vi "Paint.lv.vi"() -> ()   [LabVIEW 2015]
uses:
  Buttons/Line.ctl
  Buttons/Rectangle.ctl
  Buttons/Triangle.ctl
  Buttons/Undo.ctl
  Buttons/Redo.ctl
  Buttons/Clear.ctl
  Graphic Objects/Graphic/Ctls/Style.ctl
  <vilib>/event_ctls.llb/eventvkey.ctl
  Graphic Objects/Canvas/Type Definitions/Status.ctl
  Graphic Objects/Graphic/Graphic.lvclass/Graphic.ctl
  Graphic Objects/Canvas/Canvas.lvclass/Canvas.ctl
  Graphic Objects/Canvas/Canvas.lvclass
  <vilib>/Utility/miscctls.llb/LVPoint32TypeDef.ctl
  Graphic Objects/Graphic/Graphic.lvclass
  Graphic Objects/Line/Line.lvclass
  Graphic Objects/Line Border/Line Border.lvclass
  Graphic Objects/Rectangle/Rectangle.lvclass
  Graphic Objects/Rectangle Border/Rectangle Border.lvclass
  Graphic Objects/Triangle/Triangle.lvclass
panel:
  in  "Listbox":i32(listbox)
  in  "Tool Box":enum32{"Line", "Rectangle", "Triangle"}(radio)
  in  "Clear":T1
  in  "Redo":T2
  in  "Undo":T3
  out "Border":picture
  out "Picture":picture
  in  "Line Type":T4(ring) caption="Line Type:"
  in  "Line Width":u8=2 caption="Line Width:" min=1 max=10 step=1
  in  "Line Color":u32(colorbox) caption="Line Color:"
  # "Paint.lv"
  # "V1.0.1"
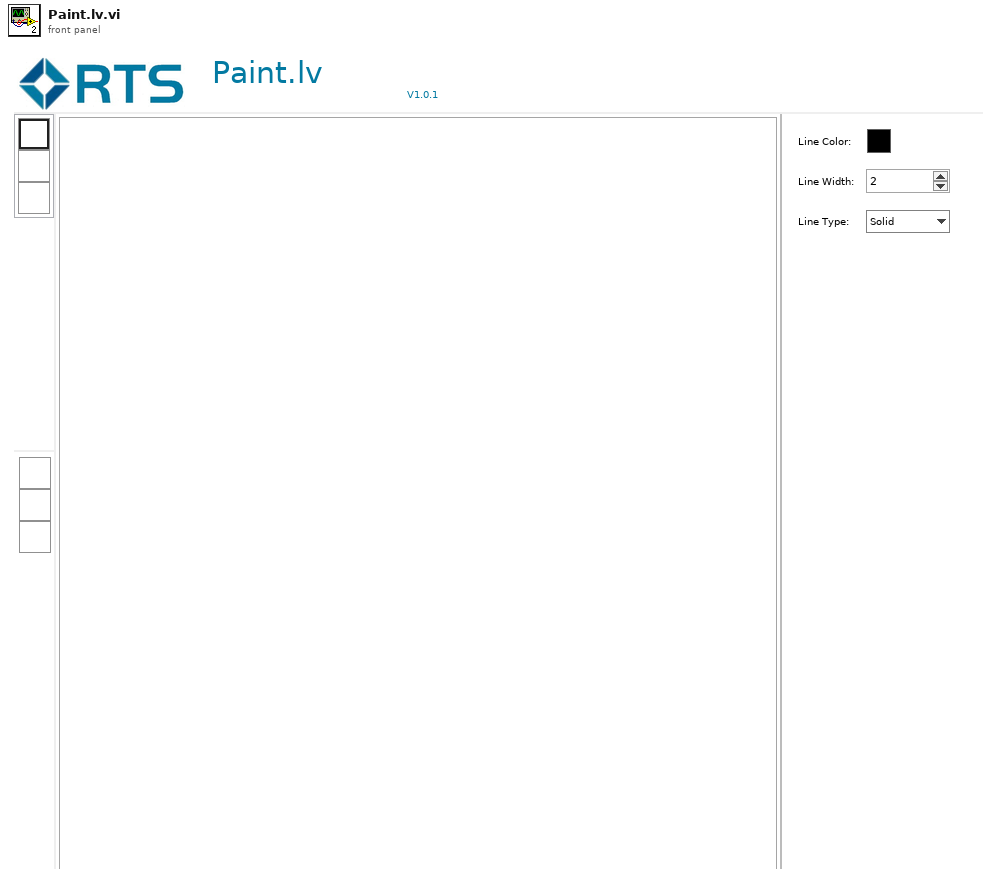
[diagram p1: front panel]
types:
  T1 = typedef "Clear.ctl" = bool
  T2 = typedef "Redo.ctl" = bool
  T3 = typedef "Undo.ctl" = bool
  T4 = enum32{"Solid", "Dash", "Dot", "DashDot", "DashDotDot"}
  T5 = typedef "Graphic.lvclass/Style.ctl" = cluster{"Color":u32, "Pen":cluster{"Width":u16, "Style":enum32{"Solid", "Dash", "Dot", "DashDot", "DashDotDot"}}}
  T6 = typedef "eventvkey.ctl" = enum16{"ASCII", "Enter", "Return", "Shift", "Ctrl", "Alt", "Cmd", "Opt", "Caps", "NumLock", "Clear", "Break", "Up", "Down", "Left", "Right", "Insert", "Delete", "Home", "End", "PageUp", "PageDown", "Escape", "Help", "Pause", "ScrollLock", "F1", "F2", "F3", "F4", "F5", "F6", "F7", "F8", "F9", "F10", "F11", "F12", "F13", "F14", "F15", "F16", "F17", "F18", "F19", "F20", "F21", "F22", "F23", "F24", "Play", "VolumeUp", "VolumeDown", "Mute", "Two Byte Char"}
  T7 = typedef "Canvas.lvclass/Status.ctl" = enum16{"Idle", "Drawing", "Modify"}
  T8 = enum32{"Invalid", "Standard", "Closed", "Hidden", "Minimized", "Maximized"}
  T9 = enum32{"invalid app kind", "Development System", "Run Time System", "Student Edition", "Embedded LabVIEW", "Evaluation", "Custom"}
  T10 = typedef "LVPoint32TypeDef.ctl" = cluster{"Horizontal":i32, "Vertical":i32}
  T11 = cluster{"Core":cluster{"Current VI Reference":refnum<vi>, "Close Panel on Exit?":bool}, "Canvas":refnum<class "Canvas.lvclass">, "MouseDown Coords":T10, "MouseUp Coords":T10, "Current Coords":T10, "Status":T7, "Drawing Graphic":refnum<class "Graphic.lvclass">, "ValidOperating":bool, "MouseDown":bool}
  T12 = cluster{"Width":u16, "Style":enum32{"Solid", "Dash", "Dot", "DashDot", "DashDotDot"}}
  T13 = cluster{"Current VI Reference":refnum<vi>, "Close Panel on Exit?":bool}
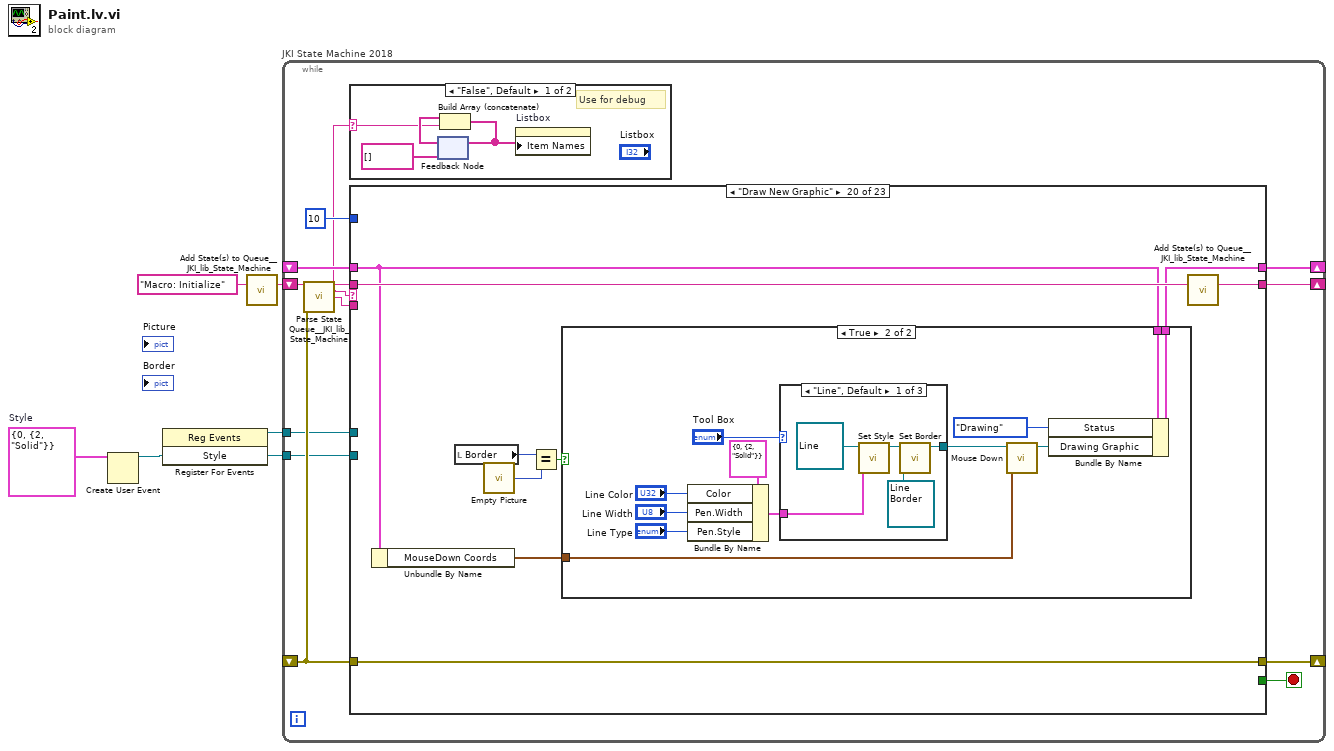
[diagram p0: block diagram]
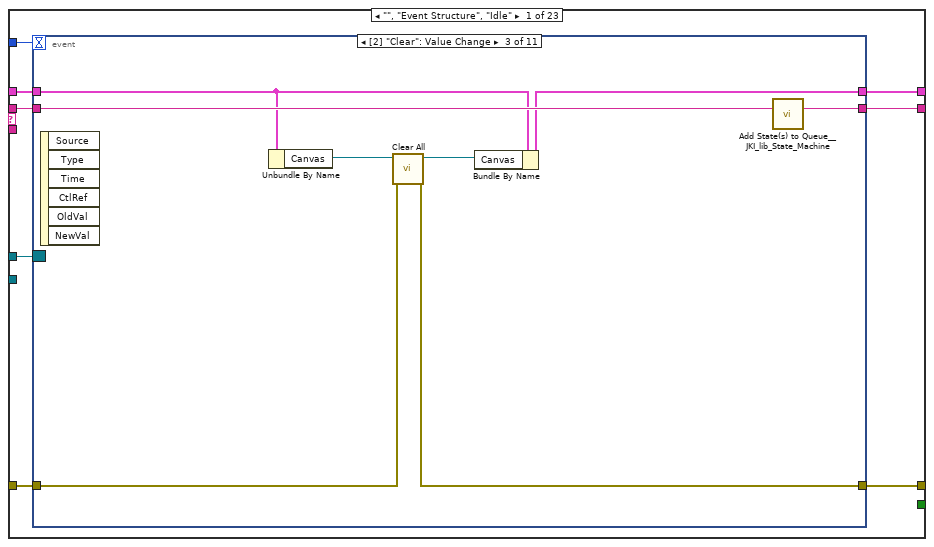
[diagram p3: hidden frame]
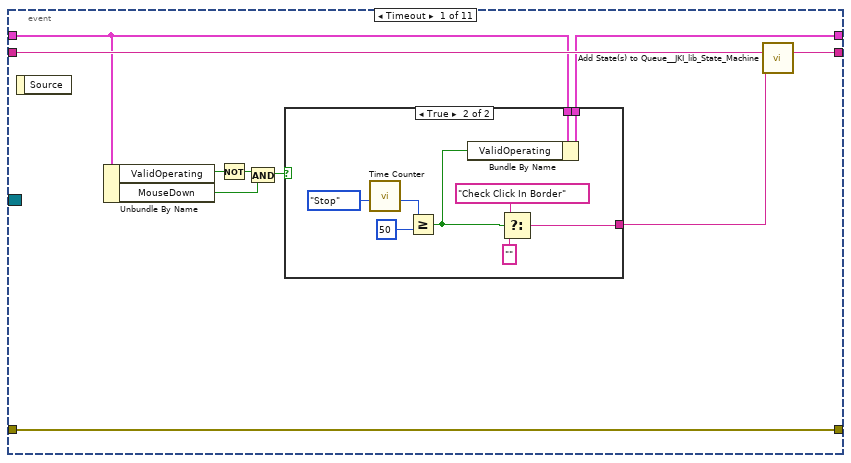
[diagram p4: hidden frame]
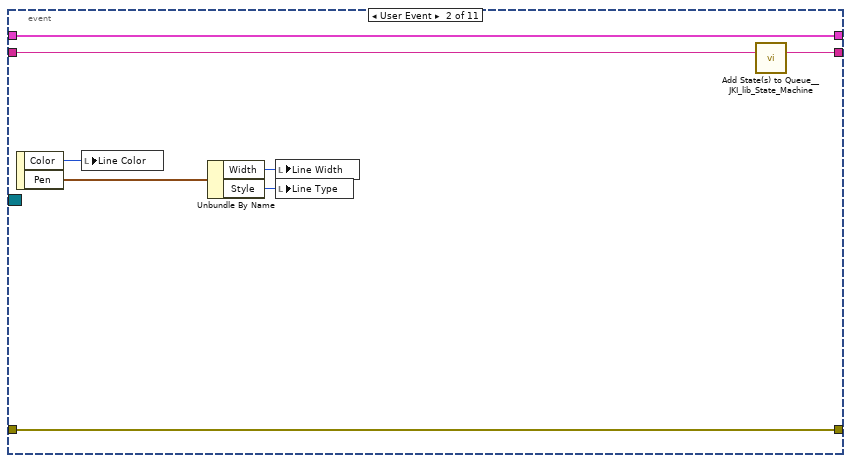
[diagram p6: hidden frame]
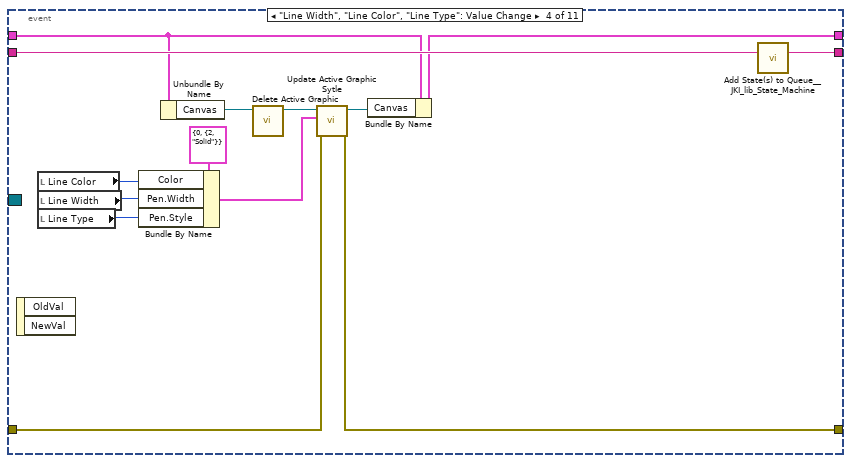
[diagram p7: hidden frame]
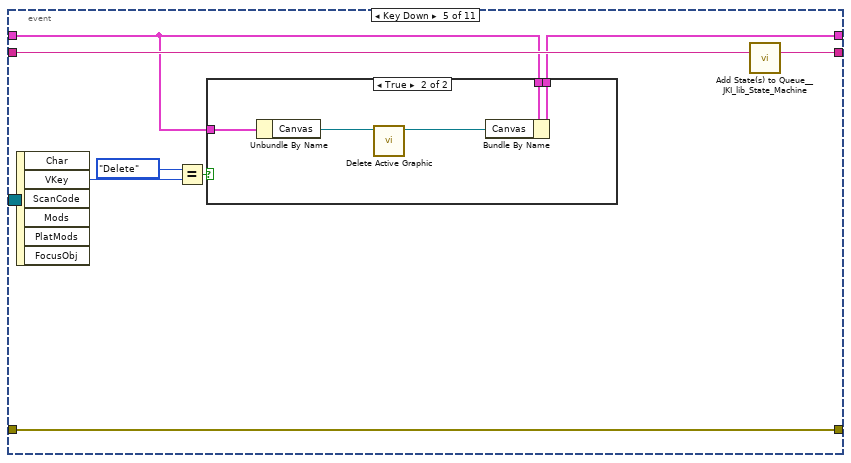
[diagram p8: hidden frame]
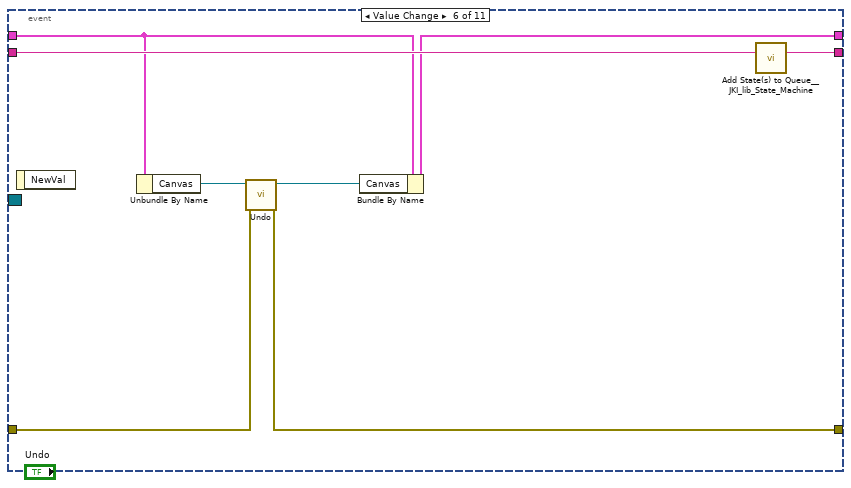
[diagram p10: hidden frame]
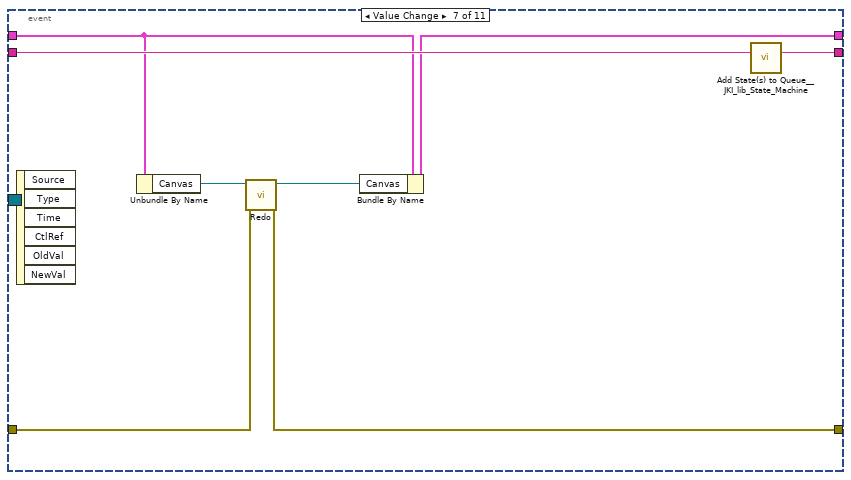
[diagram p11: hidden frame]
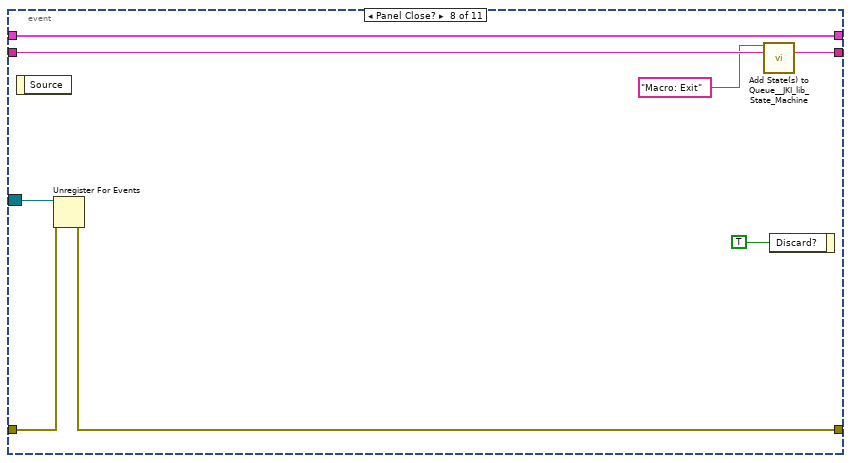
[diagram p12: hidden frame]
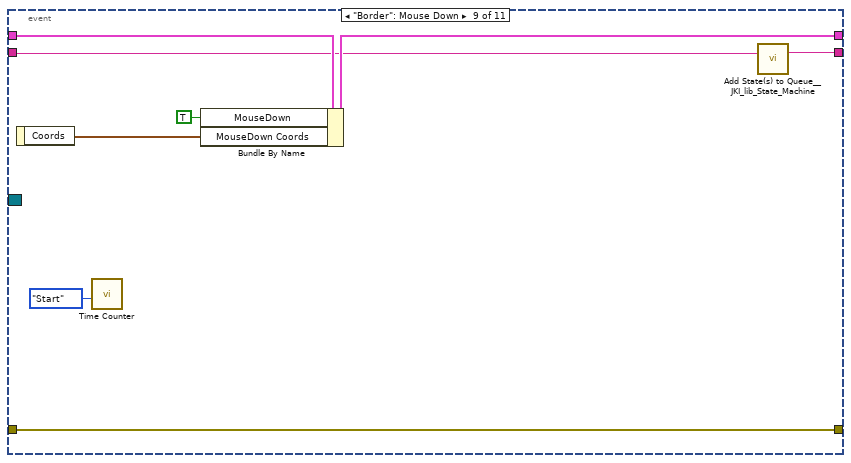
[diagram p13: hidden frame]
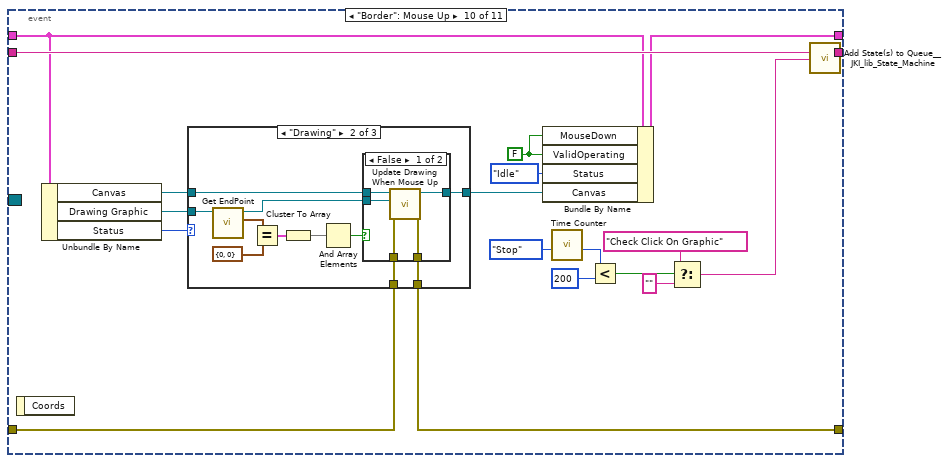
[diagram p14: hidden frame]
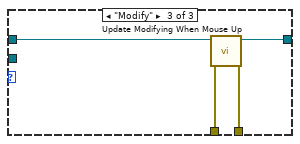
[diagram p17: hidden frame]
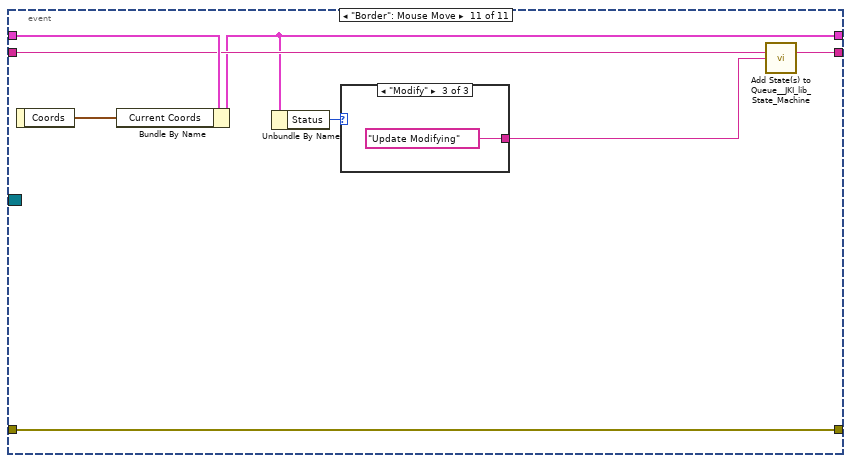
[diagram p18: hidden frame]
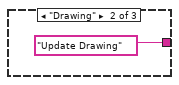
[diagram p20: hidden frame]
diagram:
  w3 = T5 {"Color"=0, "Pen"={"Width"=2, "Style"=enum."Solid"}}  # Style
  n1 = Create User Event(user event datatype=w3) -> (user event=w2:refnum<user-event>)  [unwired: 1 in, 1 out]
  n2 = register-events(w2) -> (reference out=w1:refnum<event-registration>)  [unwired: 2 in, 1 out]
  n3 = call <vilib>:"Add State(s) to Queue__JKI_lib_State_Machine.vi"("State(s) in (\"\")"="Macro: Initialize") -> ("States Out"=w4:string)  [unwired: 14 in]
  n4 = while "JKI State Machine 2018" {
    shift-right: [w12] -> _
    shift-left: _ -> [w11]
    shift-right: [w15] -> _
    shift-left: _ -> [w9]
    shift-right: [w14] -> _
    shift-left: w4 -> [w16]
    tunnel: w2 -> [w7]
    tunnel: w1 -> [w6]
    stop <- w13 stop-if-true
    n5 = call <vilib>:"Parse State Queue__JKI_lib_State_Machine.vi"("State Queue"=w16, "Error In (no error)"=w9) -> ("Remaining States"=w18:string, "Current State"=w8:string, "Arguments"=w17:string)  [unwired: 11 in]
    n6 = case shown="\"False\", Default" w8 {
      selector: w8 -> [w19 _]
      frame "False", Default {
        # "Use for debug"
        n7 = feedback #1(string[] []) -> (w21:string[])
        n8 = Build Array (concatenate)(w21, w19) -> (w20:string[])
        n9 = feedback-in #1(w20) -> ()
        n10 = property on="Listbox" class="LstBox (strict)"("Item Names"=w20) -> ()  [unwired: 2 in, 2 out]
      }
      frame "" {
      }
    }
    n11 = case shown="\"Draw New Graphic\"" w8 {
      selector: w8 -> [_ _ w185 _ _ _ _ _ _ _ _ _ _ _ _ _ _ _ _ _ _ _ _]
      tunnel: w18 -> [w30 w184 w189 w208 w214 w229 w233 w246 w252 w256 w287 w293 w304 w373 w378 w388 w392 w403 w414 w423 w459 w472 w482]
      tunnel: w17 -> [_ _ _ _ _ _ _ _ _ _ _ w288 w298 _ _ _ _ _ _ _ _ _ _]
      tunnel: w11 -> [w29 w181 w187 w201 w211 w225 w230 _ w247 w253 w284 w291 w300 w370 w375 w385 w389 w401 w412 w419 w454 w470 w479]
      tunnel: [w28 w182 w191 w205 errorcluster {"status"=FALSE, "code"=0, "source"=""} ("error out") w227 w231 w243 w248 w254 w285 w289 w301 w371 w376 w386 w390 w393 w409 w421 w457 w464 w480] -> w15
      tunnel: w9 -> [w27 w182 w190 w205 w210 w227 w231 w243 w249 w254 w285 w290 w302 w371 w376 w386 w390 w394 w410 w421 w457 w465 w480]
      tunnel: [w24 w183 w188 w207 w213 w228 w232 w245 w251 w255 w286 w292 w303 w372 w377 w387 w391 w402 w413 w422 w458 w471 w481] -> w14
      tunnel: [_ _ _ _ _ TRUE _ _ _ _ _ _ _ _ _ _ _ _ _ _ _ _ _] -> w13
      tunnel: [w26 w181 w187 w206 w211 w225 w230 w244 w247 w253 w283 w291 w300 w370 w375 w385 w389 w400 w408 w420 w456 w468 w476] -> w12
      tunnel: 10 ("Timeout") -> [w25 _ _ _ _ _ _ _ _ _ _ _ _ _ _ _ _ _ _ _ _ _ _]
      tunnel: w7 -> [_ _ _ _ _ _ _ _ _ _ w257 _ _ _ _ _ _ _ _ _ _ _ _]
      tunnel: w6 -> [w23 _ _ _ _ _ _ _ _ _ _ _ _ _ _ _ _ _ _ _ _ _ _]
      frame "", "Event Structure", "Idle" {
        n12 = event shown="[2] \"Clear\": Value Change" {
          selector: w23 -> [_ _ _ _ _ _ _ w114 _ _ _]
          dyn-events: _ -> [_ _ _ _ _ _ _ _ _ _ _]
          timeout: w25 -> [_ _ _ _ _ _ _ _ _ _ _]
          tunnel: w30 -> [w39 w57 w66 w80 w87 w102 w110 w116 w121 w146 w175]
          tunnel: w29 -> [w32 w55 w64 w78 w82 w100 w108 w119 w125 w142 w178]
          tunnel: [w40 w58 w59 w73 w88 w95 w103 w112 w127 w129 w177] -> w28
          tunnel: w27 -> [w40 w58 w60 w74 w88 w96 w104 w113 w127 w130 w177]
          tunnel: [w31 w55 w63 w77 w81 w99 w107 w119 w124 w144 w173] -> w26
          tunnel: [w38 w56 w65 w79 w86 w101 w109 w117 w122 w145 w176] -> w24
          event Timeout {
            n13 = event-data() -> ()  [unwired: 1 in, 1 out]
            n14 = Unbundle By Name(w32) -> ("ValidOperating"=w36:bool, "MouseDown"=w34:bool)
            n15 = Not(x=w36) -> (.not. x?=w35:bool)
            n16 = And(x=w35, y=w34) -> (x .and. y?=w33:bool)
            n17 = case shown="True" w33 {
              tunnel: [_ w45] -> w37
              tunnel: w32 -> [w41 w43]
              tunnel: [w41 w42] -> w31
              frame False {
              }
              frame True {
                n18 = call "Time Counter.vi"("Action"=enum16{"Start", "Stop"}."Stop") -> ("Elapsed"=w49:u32)  [unwired: 10 in]
                n19 = Greater Or Equal?(x=w49, y=u32 50) -> (x >= y?=w44:bool)
                n20 = Bundle By Name(cluster=w43, "ValidOperating"=w44) -> (w42:T11)
                n21 = Select(t="Check Click In Border", s=w44, f="") -> (s? t:f=w45:string)
              }
            }
            n22 = call <vilib>:"Add State(s) to Queue__JKI_lib_State_Machine.vi"("State(s) in (\"\")"=w39, "State(s) at Back (\"\")"=w37) -> ("States Out"=w38:string)  [unwired: 13 in]
            n23 = call <vilib>:"Add State(s) to Queue__JKI_lib_State_Machine.vi"() -> ()  [unwired: 15 in, 1 out]
          }
          event User Event {
            n24 = event-data() -> ("Color"=w54:u32, "Pen"=w53:T12)  [unwired: 1 in]
            n25 = local write "Line Color"(w54) -> ()
            n26 = Unbundle By Name(w53) -> ("Width"=w51:u16, "Style"=w52:T4)
            n27 = local write "Line Width"(w51) -> ()
            n28 = local write "Line Type"(w52) -> ()
            n29 = call <vilib>:"Add State(s) to Queue__JKI_lib_State_Machine.vi"("State(s) in (\"\")"=w57) -> ("States Out"=w56:string)  [unwired: 14 in]
            n30 = call <vilib>:"Add State(s) to Queue__JKI_lib_State_Machine.vi"() -> ()  [unwired: 15 in, 1 out]
          }
          event Value Change {
            n31 = event-data() -> ()  [unwired: 1 in, 6 out]
            n32 = Unbundle By Name(w64) -> ("Canvas"=w62:refnum<class "Canvas.lvclass">)
            n33 = call "Clear All.vi"("error in (no error)"=w60, "Canvas in"=w62) -> ("error out"=w59:errorcluster, "Canvas out"=w61:refnum<class "Canvas.lvclass">)  [unwired: 8 in]
            n34 = Bundle By Name(cluster=w64, "Canvas"=w61) -> (w63:T11)
            n35 = call <vilib>:"Add State(s) to Queue__JKI_lib_State_Machine.vi"("State(s) in (\"\")"=w66) -> ("States Out"=w65:string)  [unwired: 14 in]
            n36 = call <vilib>:"Add State(s) to Queue__JKI_lib_State_Machine.vi"() -> ()  [unwired: 15 in, 1 out]
          }
          event "Line Width", "Line Color", "Line Type": Value Change {
            n37 = event-data() -> ()  [unwired: 1 in, 2 out]
            n38 = local read "Line Color"() -> (w71:u32)
            n39 = local read "Line Width"() -> (w68:u8)
            n40 = local read "Line Type"() -> (w67:T4)
            n41 = Bundle By Name(cluster=T5 {"Color"=0, "Pen"={"Width"=2, "Style"=enum."Solid"}} ("Style"), "Color"=w71, "Pen.Width"=w68, "Pen.Style"=w67) -> (w70:T5)
            n42 = Unbundle By Name(w78) -> ("Canvas"=w76:refnum<class "Canvas.lvclass">)
            n43 = call "Delete Active Graphic.vi"("Canvas in"=w76) -> ("Canvas out"=w69:refnum<class "Canvas.lvclass">)  [unwired: 9 in, 1 out]
            n44 = call "Update Active Graphic Sytle.vi"("error in (no error)"=w74, "Style"=w70, "Canvas in"=w69) -> ("error out"=w73:errorcluster, "Canvas out"=w75:refnum<class "Canvas.lvclass">)  [unwired: 7 in]
            n45 = Bundle By Name(cluster=w78, "Canvas"=w75) -> (w77:T11)
            n46 = call <vilib>:"Add State(s) to Queue__JKI_lib_State_Machine.vi"("State(s) in (\"\")"=w80) -> ("States Out"=w79:string)  [unwired: 14 in]
            n47 = call <vilib>:"Add State(s) to Queue__JKI_lib_State_Machine.vi"() -> ()  [unwired: 15 in, 1 out]
          }
          event Key Down {
            n48 = event-data() -> ("VKey"=w85:T6)  [unwired: 1 in, 5 out]
            n49 = Equal?(x=eventvkey."Delete" ("VKey"), y=w85) -> (x = y?=w83:bool)
            n50 = case shown="True" w83 {
              tunnel: w82 -> [_ w94]
              tunnel: w82 -> [w89 w91]
              tunnel: [w89 w90] -> w81
              frame False {
              }
              frame True {
                n51 = Unbundle By Name(w94) -> ("Canvas"=w93:refnum<class "Canvas.lvclass">)
                n52 = call "Delete Active Graphic.vi"("Canvas in"=w93) -> ("Canvas out"=w92:refnum<class "Canvas.lvclass">)  [unwired: 9 in, 1 out]
                n53 = Bundle By Name(cluster=w91, "Canvas"=w92) -> (w90:T11)
              }
            }
            n54 = call <vilib>:"Add State(s) to Queue__JKI_lib_State_Machine.vi"("State(s) in (\"\")"=w87) -> ("States Out"=w86:string)  [unwired: 14 in]
            n55 = call <vilib>:"Add State(s) to Queue__JKI_lib_State_Machine.vi"() -> ()  [unwired: 15 in, 1 out]
          }
          event Value Change {
            n56 = event-data() -> ()  [unwired: 1 in, 1 out]
            n57 = Unbundle By Name(w100) -> ("Canvas"=w98:refnum<class "Canvas.lvclass">)
            n58 = call "Undo.vi"("error in (no error)"=w96, "Canvas in"=w98) -> ("error out"=w95:errorcluster, "Canvas out"=w97:refnum<class "Canvas.lvclass">)  [unwired: 8 in]
            n59 = Bundle By Name(cluster=w100, "Canvas"=w97) -> (w99:T11)
            n60 = call <vilib>:"Add State(s) to Queue__JKI_lib_State_Machine.vi"("State(s) in (\"\")"=w102) -> ("States Out"=w101:string)  [unwired: 14 in]
            n61 = call <vilib>:"Add State(s) to Queue__JKI_lib_State_Machine.vi"() -> ()  [unwired: 15 in, 1 out]
          }
          event Value Change {
            n62 = event-data() -> ()  [unwired: 1 in, 6 out]
            n63 = Unbundle By Name(w108) -> ("Canvas"=w106:refnum<class "Canvas.lvclass">)
            n64 = call "Redo.vi"("error in (no error)"=w104, "Canvas in"=w106) -> ("error out"=w103:errorcluster, "Canvas out"=w105:refnum<class "Canvas.lvclass">)  [unwired: 8 in]
            n65 = Bundle By Name(cluster=w108, "Canvas"=w105) -> (w107:T11)
            n66 = call <vilib>:"Add State(s) to Queue__JKI_lib_State_Machine.vi"("State(s) in (\"\")"=w110) -> ("States Out"=w109:string)  [unwired: 14 in]
            n67 = call <vilib>:"Add State(s) to Queue__JKI_lib_State_Machine.vi"() -> ()  [unwired: 15 in, 1 out]
          }
          event Panel Close? {
            (unwired) TRUE ("Discard?")
            n68 = event-data() -> ()  [unwired: 1 in, 1 out]
            n69 = Unregister For Events(event registration refnum=w114, error in=w113) -> (error out=w112:errorcluster)
            n70 = call <vilib>:"Add State(s) to Queue__JKI_lib_State_Machine.vi"("State(s) in Front (\"\")"="Macro: Exit", "State(s) in (\"\")"=w116) -> ("States Out"=w117:string)  [unwired: 13 in]
            n71 = event-data("Discard?"=TRUE) -> ()  [unwired: 1 in, 1 out]
            n72 = call <vilib>:"Add State(s) to Queue__JKI_lib_State_Machine.vi"("State(s) in Front (\"\")"="Macro: Exit") -> ()  [unwired: 14 in, 1 out]
          }
          event "Border": Mouse Down {
            n73 = event-data() -> ("Coords"=w123:T10)  [unwired: 1 in]
            n74 = call "Time Counter.vi"("Action"=enum16{"Start", "Stop"}."Start") -> ()  [unwired: 10 in, 1 out]
            n75 = Bundle By Name(cluster=w125, "MouseDown"=TRUE, "MouseDown Coords"=w123) -> (w124:T11)
            n76 = call <vilib>:"Add State(s) to Queue__JKI_lib_State_Machine.vi"("State(s) in (\"\")"=w121) -> ("States Out"=w122:string)  [unwired: 14 in]
            n77 = call <vilib>:"Add State(s) to Queue__JKI_lib_State_Machine.vi"() -> ()  [unwired: 15 in, 1 out]
          }
          event "Border": Mouse Up {
            w128 = FALSE ("ValidOperating")
            n78 = event-data() -> ()  [unwired: 1 in, 1 out]
            n79 = Unbundle By Name(w142) -> ("Canvas"=w139:refnum<class "Canvas.lvclass">, "Drawing Graphic"=w140:refnum<class "Graphic.lvclass">, "Status"=w141:T7)
            n80 = case shown="\"Drawing\"" w141 {
              tunnel: w140 -> [_ w157 _]
              tunnel: w139 -> [w148 w159 w170]
              tunnel: [w148 w158 w169] -> w138
              tunnel: w130 -> [w147 w150 w168]
              tunnel: [w147 w149 w167] -> w129
              frame "Idle", Default {
              }
              frame "Drawing" {
                n81 = call "Get EndPoint.vi"("Graphic in"=w157) -> ("EndPoint"=w155:cluster{"x":i16, "y":i16}, "Graphic out"=w156:refnum<class "Graphic.lvclass">)  [unwired: 8 in, 1 out]
                n82 = Equal?(x=w155, y=cluster{"x":i16, "y":i16} {"x"=0, "y"=0} ("EndPoint")) -> (x = y?=w153:cluster{"x":bool, "y":bool})
                n83 = Cluster To Array(cluster=w153) -> (array=w152:bool[])
                n84 = And Array Elements(Boolean array=w152) -> (logical AND=w151:bool)
                n85 = case shown="False" w151 {
                  tunnel: w159 -> [w164 w166]
                  tunnel: [w163 w166] -> w158
                  tunnel: w156 -> [w162 _]
                  tunnel: w150 -> [w161 w165]
                  tunnel: [w160 w165] -> w149
                  frame False {
                    n86 = call "Update Drawing When Mouse Up.vi"("error in (no error)"=w161, "Graphic"=w162, "Canvas in"=w164) -> ("error out"=w160:errorcluster, "Canvas out"=w163:refnum<class "Canvas.lvclass">)  [unwired: 7 in]
                  }
                  frame True {
                  }
                }
              }
              frame "Modify" {
                n87 = call "Update Modifying When Mouse Up.vi"("error in (no error)"=w168, "Canvas in"=w170) -> ("error out"=w167:errorcluster, "Canvas out"=w169:refnum<class "Canvas.lvclass">)  [unwired: 8 in]
              }
            }
            n88 = Bundle By Name(cluster=w142, "MouseDown"=w128, "ValidOperating"=w128, "Status"=Status."Idle", "Canvas"=w138) -> (w144:T11)
            n89 = call "Time Counter.vi"("Action"=enum16{"Start", "Stop"}."Stop") -> ("Elapsed"=w136:u32)  [unwired: 10 in]
            n90 = Less?(x=w136, y=u32 200) -> (x < y?=w134:bool)
            n91 = Select(t="Check Click On Graphic", s=w134, f="") -> (s? t:f=w131:string)
            n92 = call <vilib>:"Add State(s) to Queue__JKI_lib_State_Machine.vi"("State(s) in (\"\")"=w146, "State(s) at Back (\"\")"=w131) -> ("States Out"=w145:string)  [unwired: 13 in]
          }
          event "Border": Mouse Move {
            n93 = event-data() -> ("Coords"=w174:T10)  [unwired: 1 in]
            n94 = Bundle By Name(cluster=w178, "Current Coords"=w174) -> (w173:T11)
            n95 = Unbundle By Name(w173) -> ("Status"=w172:T7)
            n96 = case shown="\"Modify\"" w172 {
              tunnel: [_ "Update Drawing" "Update Modifying"] -> w171
              frame "Idle", Default {
              }
              frame "Drawing" {
              }
              frame "Modify" {
              }
            }
            n97 = call <vilib>:"Add State(s) to Queue__JKI_lib_State_Machine.vi"("State(s) in (\"\")"=w175, "State(s) at Back (\"\")"=w171) -> ("States Out"=w176:string)  [unwired: 13 in]
            n98 = call <vilib>:"Add State(s) to Queue__JKI_lib_State_Machine.vi"() -> ()  [unwired: 15 in, 1 out]
          }
        }
      }
      frame "---------- Core ----------" {
        # "Do not put any code in this frame.\n(it is a separator no-op)"
        n99 = call <vilib>:"Add State(s) to Queue__JKI_lib_State_Machine.vi"("State(s) in (\"\")"=w184) -> ("States Out"=w183:string)  [unwired: 14 in]
      }
      frame Default {
        w194 = 42 items=["No error", "Argument error", "Memory is full", "Out of zone", "End of file", "File already open", "Generic file I/O error", "File not found", "File permission error", "Disk is full", "Duplicate path", "Too many files open", "System feature not enabled", "Resource file not found", "Cannot add resource", "Resource not found", "Image not found", "Image memory error", "Pen does not exist", "Config type invalid", "Config token not found", "Config parse error", "Config memory error", "Bad external code format", "Bad external code offset", "External code not present", "Null window", "Destroy window error", "Null menu", "Print aborted", "Bad print record", "Print driver error", "Windows error during printing", "Memory error during printing", "Print dialog error", "Generic print error", "Invalid device refnum", "Device not found", "Device parameter error", "Device unit error", "Cannot open device", "Device call aborted", "Generic error", "Cancelled by user", "Object ID too low", "Object ID too high", "Object not in heap", "Unknown heap", "Unknown object (invalid DefProc)", "Unknown object (DefProc not in table)", "Message out of range", "Invalid (null) method", "Unknown message", "Manager call not supported", "Bad address", "Network operation in progress", "Network operation timed out", "Connection is busy", "Network attribute not supported", "Network error", "Address in use", "System out of memory", "Connection aborted", "Connection refused", "Not connected", "Already connected", "Connection closed", "Initialization error (interapplication manager)", "Bad occurrence", "Wait on unbound occurrence handler", "Occurrence queue overflow", "Datalog type conflict", "Unused", "Unrecognized type (interapplication manager)", "Memory corrupt", "Failed to make temporary DLL", "Old CIN version", "Drag socket not found", "Failed to load drop-object", "Failed to register OLE object", "Failed to release OLE object", "Format specifier type mismatch", "Unknown format specifier", "Too few format specifiers", "Too many format specifiers", "Scan failed", "Newer CIN version", "Error converting to variant", "Runtime menu error", "Password tampered", "Variant attribute not found", "Incompatible variant data type", "Event data is not available", "Event Store is not present", "Occurrence is not found", "Event Queue is not created", "Event info is not available", "Refnum passed is NULL", "Error retrieving Class GUID", "Error retrieving CoClass GUID", "Error retrieving TypeLib GUID.", "Bad built application magic bytes.", "Specific driver is different from the specific driver associated with the Logical Name.", "There is no session opened to the class driver.", "Max Error", "MAX - Error with config objects", "MAX - Error loading configuration", "MAX - Group not supported"]
        # "Current State"
        # "Do not delete, rename, or modify this frame.\n(this is used to capture unhandled states and typos)"
        # "Handle mistyped state name (developer tool)"
        n100 = Format Into String(format string="Software Exception: Unhandled State \"%s\"." ("message"), error in=w190, w185) -> (resulting string=w193:string, error out=w192:errorcluster)  [unwired: 1 in]
        n101 = call <vilib>:"Error Cluster From Error Code.vi"("show call chain? (False)"=TRUE, "error in (no error)"=w192, "error message (\"\")"=w193, "error code (0)"=w194) -> ("error out"=w191:errorcluster)  [unwired: 5 in]
        n102 = call <vilib>:"Add State(s) to Queue__JKI_lib_State_Machine.vi"("State(s) in (\"\")"=w189) -> ("States Out"=w188:string)  [unwired: 14 in]
      }
      frame "Initialize Core Data" {
        # "Do not delete, rename, or modify this frame.\n(this is used to determine panel behavior on exit)"
        # "originally closed?"
        # "exe?"
        # "If panel starts closed or is an EXE, then close it when we exit"
        n103 = property class="VI"() -> ("FP.State"=w198:T8)  [unwired: 2 in, 2 out]
        n104 = property class="App"() -> ("App.Kind"=w204:T9)  [unwired: 2 in, 2 out]
        n105 = control-ref of="Current VI Reference"() -> (w199:refnum<vi>)
        n106 = Equal?(x=w198, y=T8."Closed" ("Front Panel Window:State")) -> (x = y?=w196:bool)
        n107 = Equal?(x=w204, y=T9."Run Time System" ("Application:Kind")) -> (x = y?=w202:bool)
        n108 = Or(x=w196, y=w202) -> (x .or. y?=w200:bool)
        n109 = Bundle By Name(cluster=w201, "Core.Current VI Reference"=w199, "Core.Close Panel on Exit?"=w200) -> (w206:T11)
        n110 = call <vilib>:"Add State(s) to Queue__JKI_lib_State_Machine.vi"("State(s) in (\"\")"=w208) -> ("States Out"=w207:string)  [unwired: 14 in]
      }
      frame "Error Handler" {
        # "Unhandled Error -- Display it"
        # "Handle any errors here.\nYou can also output any states to clean-up after errors occur"
        # "Clear error"
        n111 = call <vilib>:"General Error Handler.vi"("error in (no error)"=w210) -> ()  [unwired: 10 in, 5 out]
        n112 = call <vilib>:"Add State(s) to Queue__JKI_lib_State_Machine.vi"("State(s) in Front (\"\")"="/* Post Error States", "State(s) in (\"\")"=w214) -> ("States Out"=w213:string)  [unwired: 13 in]
      }
      frame "Exit" {
        n113 = Unbundle By Name(w225) -> ("Canvas"=w224:refnum<class "Canvas.lvclass">)
        n114 = call "Get PicUndo Queue.vi"("Canvas in"=w224) -> ("Undo Queue"=w222:refnum<queue>, "Canvas out"=w223:refnum<class "Canvas.lvclass">)  [unwired: 8 in, 1 out]
        n115 = Release Queue(queue=w222) -> ()  [unwired: 2 in, 3 out]
        n116 = call "Get PicRedo Queue.vi"("Canvas in"=w223) -> ("PicRedo Queue"=w221:refnum<queue>, "Canvas out"=w219:refnum<class "Canvas.lvclass">)  [unwired: 8 in, 1 out]
        n117 = Release Queue(queue=w221) -> ()  [unwired: 2 in, 3 out]
        n118 = call "Get GraphicsUndo.vi"("Canvas in"=w219) -> ("GraphicsUndo"=w218:refnum<queue>, "Canvas out"=w220:refnum<class "Canvas.lvclass">)  [unwired: 8 in, 1 out]
        n119 = Release Queue(queue=w218) -> ()  [unwired: 2 in, 3 out]
        n120 = call "Get GraphicsRedo.vi"("Canvas in"=w220) -> ("GraphicsRedo"=w217:refnum<queue>, "Canvas out"=w216:refnum<class "Canvas.lvclass">)  [unwired: 8 in, 1 out]
        n121 = Release Queue(queue=w217) -> ()  [unwired: 2 in, 3 out]
        n122 = call "Get UpdateSytle Event.vi"("Canvas in"=w216) -> ("UpdateSytle Event"=w215:refnum<user-event>)  [unwired: 8 in, 2 out]
        n123 = Destroy User Event(user event=w215) -> ()  [unwired: 1 in, 1 out]
        n124 = call <vilib>:"Add State(s) to Queue__JKI_lib_State_Machine.vi"("State(s) in (\"\")"=w229) -> ("States Out"=w228:string)  [unwired: 14 in]
      }
      frame "---------- Data ----------" {
        # "Do not put any code in this frame.\n(It is a separator no-op. You can make a copy of this frame to create a new Data frame)"
        n125 = call <vilib>:"Add State(s) to Queue__JKI_lib_State_Machine.vi"("State(s) in (\"\")"=w233) -> ("States Out"=w232:string)  [unwired: 14 in]
      }
      frame "Data: Initialize" {
        w234 = FALSE  # MouseDown
        w235 = FALSE  # ValidOperating
        w236 = refnum<class "Graphic.lvclass"> refnum  # Drawing Graphic
        w237 = Status."Idle"  # Status
        w238 = T10 {"Horizontal"=0, "Vertical"=0}  # Current Coords
        w239 = T10 {"Horizontal"=0, "Vertical"=0}  # MouseUp Coords
        w240 = T10 {"Horizontal"=0, "Vertical"=0}  # MouseDown Coords
        w241 = refnum<class "Canvas.lvclass"> refnum  # Canvas
        w242 = T13 {"Current VI Reference"=refnum, "Close Panel on Exit?"=FALSE}  # Core
        n126 = Bundle("Core"=w242, "Canvas"=w241, "MouseDown Coords"=w240, "MouseUp Coords"=w239, "Current Coords"=w238, "Status"=w237, "Drawing Graphic"=w236, "ValidOperating"=w235, "MouseDown"=w234) -> (w244:T11)  [unwired: 1 in]
        n127 = call <vilib>:"Add State(s) to Queue__JKI_lib_State_Machine.vi"("State(s) in (\"\")"=w246) -> ("States Out"=w245:string)  [unwired: 14 in]
      }
      frame "Data: Cleanup" {
        n128 = Unbundle By Name(w247) -> ("Core.Current VI Reference"=w250:refnum<vi>)
        n129 = Close Reference(reference=w250, error in (no error)=w249) -> (error out=w248:errorcluster)
        n130 = call <vilib>:"Add State(s) to Queue__JKI_lib_State_Machine.vi"("State(s) in (\"\")"=w252) -> ("States Out"=w251:string)  [unwired: 14 in]
      }
      frame "---------- UI ----------" {
        n131 = call <vilib>:"Add State(s) to Queue__JKI_lib_State_Machine.vi"("State(s) in (\"\")"=w256) -> ("States Out"=w255:string)  [unwired: 14 in]
      }
      frame "UI: Initialize" {
        w267 = refnum<class "Graphic.lvclass">[] []
        n132 = Unbundle By Name(w284) -> ("Canvas"=w275:refnum<class "Canvas.lvclass">)
        n133 = control-ref of="Border"() -> (w270:refnum<vi>)
        n134 = control-ref of="Picture"() -> (w271:refnum<vi>)
        n135 = Obtain Queue(name (unnamed)="PicUndo", element data type=picture data[5B] ("Border")) -> (queue out=w273:refnum<queue>)  [unwired: 3 in, 2 out]
        n136 = Obtain Queue(name (unnamed)="PicRedo", element data type=picture data[5B] ("Border")) -> (queue out=w272:refnum<queue>)  [unwired: 3 in, 2 out]
        n137 = Obtain Queue(name (unnamed)="GraphicsRedo", element data type=w267) -> (queue out=w263:refnum<queue>)  [unwired: 3 in, 2 out]
        n138 = Obtain Queue(name (unnamed)="GraphicsUndo", element data type=w267) -> (queue out=w264:refnum<queue>)  [unwired: 3 in, 2 out]
        n139 = call "Set picUndo Queue.vi"("Undo Queue"=w273, "Canvas in"=w275) -> ("Canvas out"=w278:refnum<class "Canvas.lvclass">)  [unwired: 8 in, 1 out]
        n140 = call "Set PicRedo Queue.vi"("PicRedo Queue"=w272, "Canvas in"=w278) -> ("Canvas out"=w277:refnum<class "Canvas.lvclass">)  [unwired: 8 in, 1 out]
        n141 = call "Set PictureRef.vi"("PictureRef"=w271, "Canvas in"=w277) -> ("Canvas out"=w276:refnum<class "Canvas.lvclass">)  [unwired: 8 in, 1 out]
        n142 = call "Set BorderRef.vi"("BorderRef"=w270, "Canvas in"=w276) -> ("Canvas out"=w274:refnum<class "Canvas.lvclass">)  [unwired: 8 in, 1 out]
        n143 = call "Set GraphicsUndo.vi"("GraphicsUndo"=w264, "Canvas in"=w274) -> ("Canvas out"=w266:refnum<class "Canvas.lvclass">)  [unwired: 8 in, 1 out]
        n144 = call "Set GraphicsRedo.vi"("GraphicsRedo"=w263, "Canvas in"=w266) -> ("Canvas out"=w265:refnum<class "Canvas.lvclass">)  [unwired: 8 in, 1 out]
        n145 = call "Clear All.vi"("Canvas in"=w265) -> ("Canvas out"=w259:refnum<class "Canvas.lvclass">)  [unwired: 9 in, 1 out]
        n146 = call "Set UpdateSytle Event.vi"("UpdateSytle Event"=w257, "Canvas in"=w259) -> ("Canvas out"=w258:refnum<class "Canvas.lvclass">)  [unwired: 8 in, 1 out]
        n147 = local write "Line Color"(u32 0 ("Line Color")) -> ()
        n148 = local write "Line Type"(T4."Solid" ("Line Type")) -> ()
        n149 = local write "Line Width"(u8 2 ("Line Width")) -> ()
        n150 = Bundle By Name(cluster=w284, "Canvas"=w258) -> (w283:T11)
        n151 = call <vilib>:"Add State(s) to Queue__JKI_lib_State_Machine.vi"("State(s) in (\"\")"=w287) -> ("States Out"=w286:string)  [unwired: 14 in]
      }
      frame "UI: Cursor Set" {
        # "Argument"
        n152 = case shown="\"Idle\", Default" w288 {
          tunnel: w290 -> [w295 w297]
          tunnel: [w294 w296] -> w289
          frame "Idle", Default {
            n153 = call <vilib>:"Unset Busy.vi"("error in (no error)"=w295) -> ("error out"=w294:errorcluster)  [unwired: 10 in]
          }
          frame "Busy" {
            n154 = call <vilib>:"Set Busy.vi"("error in (no error)"=w297) -> ("error out"=w296:errorcluster)  [unwired: 9 in, 1 out]
          }
        }
        n155 = call <vilib>:"Add State(s) to Queue__JKI_lib_State_Machine.vi"("State(s) in (\"\")"=w293) -> ("States Out"=w292:string)  [unwired: 14 in]
      }
      frame "UI: Front Panel State" {
        # "Argument"
        n156 = Unbundle By Name(w300) -> ("Core.Current VI Reference"=w299:refnum<vi>)
        n157 = case shown="\"Minimize\", \"Minimized\"" w298 {
          tunnel: w302 -> [w310 w325 w336 w349 w362]
          tunnel: [w312 w326 w338 w351 w364] -> w301
          tunnel: w299 -> [w311 w323 w337 w350 w363]
          frame "Open", "Standard", Default {
            w305 = T8."Standard" ("State")
            n158 = property class="VI"(reference=w311, error in=w310) -> (reference out=w308:refnum<vi>, error out=w309:errorcluster, "FP.State"=w307:T8)
            n159 = Not Equal?(x=w307, y=w305) -> (x != y?=w306:bool)
            n160 = case shown="True" w306 {
              tunnel: [w316 w318] -> w312
              tunnel: w309 -> [w315 w318]
              tunnel: w308 -> [w314 _]
              tunnel: w305 -> [w313 _]
              frame True {
                n161 = invoke class="VI" method="FP.Open"(reference=w314, error in=w315, "Activate"=TRUE, "State"=w313) -> (error out=w316:errorcluster)  [unwired: 1 in, 4 out]
              }
              frame False {
              }
            }
          }
          frame "Close", "Closed" {
            n162 = property class="VI"(reference=w323, error in=w325) -> (reference out=w322:refnum<vi>, error out=w324:errorcluster, "FP.State"=w320:T8)
            n163 = Not Equal?(x=w320, y=T8."Closed" ("Front Panel Window:State")) -> (x != y?=w319:bool)
            n164 = case shown="True" w319 {
              tunnel: [w327 w330] -> w326
              tunnel: w324 -> [w327 w329]
              tunnel: w322 -> [_ w328]
              frame False {
              }
              frame True {
                n165 = invoke class="VI" method="FP.Close"(reference=w328, error in=w329) -> (error out=w330:errorcluster)  [unwired: 1 in, 2 out]
              }
            }
          }
          frame "Hidden", "Hide" {
            w331 = T8."Hidden" ("State")
            n166 = property class="VI"(reference=w337, error in=w336) -> (reference out=w334:refnum<vi>, error out=w335:errorcluster, "FP.State"=w333:T8)
            n167 = Not Equal?(x=w333, y=w331) -> (x != y?=w332:bool)
            n168 = case shown="True" w332 {
              tunnel: [w342 w343] -> w338
              tunnel: w335 -> [w341 w343]
              tunnel: w334 -> [w340 _]
              tunnel: w331 -> [w339 _]
              frame True {
                n169 = invoke class="VI" method="FP.Open"(reference=w340, error in=w341, "State"=w339) -> (error out=w342:errorcluster)  [unwired: 2 in, 4 out]
              }
              frame False {
              }
            }
          }
          frame "Minimize", "Minimized" {
            w344 = T8."Minimized" ("State")
            n170 = property class="VI"(reference=w350, error in=w349) -> (reference out=w347:refnum<vi>, error out=w348:errorcluster, "FP.State"=w346:T8)
            n171 = Not Equal?(x=w346, y=w344) -> (x != y?=w345:bool)
            n172 = case shown="True" w345 {
              tunnel: [w355 w356] -> w351
              tunnel: w348 -> [w354 w356]
              tunnel: w347 -> [w353 _]
              tunnel: w344 -> [w352 _]
              frame True {
                n173 = invoke class="VI" method="FP.Open"(reference=w353, error in=w354, "State"=w352) -> (error out=w355:errorcluster)  [unwired: 2 in, 4 out]
              }
              frame False {
              }
            }
          }
          frame "Maximize", "Maximized" {
            w357 = T8."Maximized" ("State")
            n174 = property class="VI"(reference=w363, error in=w362) -> (reference out=w360:refnum<vi>, error out=w361:errorcluster, "FP.State"=w359:T8)
            n175 = Not Equal?(x=w359, y=w357) -> (x != y?=w358:bool)
            n176 = case shown="True" w358 {
              tunnel: [w368 w369] -> w364
              tunnel: w361 -> [w367 w369]
              tunnel: w360 -> [w366 _]
              tunnel: w357 -> [w365 _]
              frame True {
                n177 = invoke class="VI" method="FP.Open"(reference=w366, error in=w367, "State"=w365) -> (error out=w368:errorcluster)  [unwired: 2 in, 4 out]
              }
              frame False {
              }
            }
          }
        }
        n178 = call <vilib>:"Add State(s) to Queue__JKI_lib_State_Machine.vi"("State(s) in (\"\")"=w304) -> ("States Out"=w303:string)  [unwired: 14 in]
      }
      frame "---------- Macro ----------" {
        n179 = call <vilib>:"Add State(s) to Queue__JKI_lib_State_Machine.vi"("State(s) in (\"\")"=w373) -> ("States Out"=w372:string)  [unwired: 14 in]
      }
      frame "Macro: Initialize" {
        w374 = "Data: Initialize\nInitialize Core Data\nUI: Initialize\nUI: Front Panel State >> Open"  # Data: Initialize Initialize Core Data UI: Initialize UI: Front Panel State >> Open
        n180 = call <vilib>:"Add State(s) to Queue__JKI_lib_State_Machine.vi"("State(s) in Front (\"\")"=w374, "State(s) in (\"\")"=w378) -> ("States Out"=w377:string)  [unwired: 13 in]
      }
      frame "Macro: Exit" {
        # "Exit Macro\n(This is called once, when the VI exits)"
        n181 = Unbundle By Name(w385) -> ("Core.Close Panel on Exit?"=w384:bool)
        n182 = Select(t="UI: Front Panel State >> Close", s=w384, f="") -> (s? t:f=w381:string)
        n183 = call <vilib>:"Add State(s) to Queue__JKI_lib_State_Machine.vi"("State(s) in (\"\")"=w381, "State(s) at Back (\"\")"="Data: Cleanup\nExit") -> ("States Out"=w379:string)  [unwired: 13 in]
        n184 = call <vilib>:"Add State(s) to Queue__JKI_lib_State_Machine.vi"("State(s) in Front (\"\")"=w379, "State(s) in (\"\")"=w388) -> ("States Out"=w387:string)  [unwired: 13 in]
      }
      frame "---------- Messages----------" {
        n185 = call <vilib>:"Add State(s) to Queue__JKI_lib_State_Machine.vi"("State(s) in (\"\")"=w392) -> ("States Out"=w391:string)  [unwired: 14 in]
      }
      frame "Update Modifying" {
        n186 = Unbundle By Name(w401) -> ("Canvas"=w397:refnum<class "Canvas.lvclass">, "Current Coords"=w399:T10, "MouseDown Coords"=w398:T10)
        n187 = Subtract(x=w399, y=w398) -> (x-y=w395:T10)
        n188 = call "Modify Selected Graphicvi.vi"("error in (no error)"=w394, "Coords"=w395, "Canvas in"=w397) -> ("error out"=w393:errorcluster, "Canvas out"=w396:refnum<class "Canvas.lvclass">)  [unwired: 7 in]
        n189 = Bundle By Name(cluster=w401, "Canvas"=w396) -> (w400:T11)
        n190 = call <vilib>:"Add State(s) to Queue__JKI_lib_State_Machine.vi"("State(s) in (\"\")"=w403) -> ("States Out"=w402:string)  [unwired: 14 in]
      }
      frame "Update Drawing" {
        n191 = Unbundle By Name(w412) -> ("Canvas"=w411:refnum<class "Canvas.lvclass">, "Drawing Graphic"=w406:refnum<class "Graphic.lvclass">, "Current Coords"=w405:T10)
        n192 = call-dynamic "Mouse Up.vi"("Point"=w405, "Graphic in"=w406) -> ("Graphic out"=w404:refnum<class "Graphic.lvclass">)  [unwired: 8 in, 1 out]
        n193 = call "Update When Mouse Move.vi"("error in (no error)"=w410, "Graphic"=w404, "Canvas in"=w411) -> ("error out"=w409:errorcluster, "Canvas out"=w407:refnum<class "Canvas.lvclass">)  [unwired: 7 in]
        n194 = Bundle By Name(cluster=w412, "Canvas"=w407, "Drawing Graphic"=w404) -> (w408:T11)
        n195 = call <vilib>:"Add State(s) to Queue__JKI_lib_State_Machine.vi"("State(s) in (\"\")"=w414) -> ("States Out"=w413:string)  [unwired: 14 in]
      }
      frame "Draw New Graphic" {
        n196 = Unbundle By Name(w419) -> ("MouseDown Coords"=w418:T10)
        n197 = local read "Border"() -> (w417:picture)
        n198 = call "Empty Picture"() -> ("empty picture"=w416:picture)
        n199 = Equal?(x=w417, y=w416) -> (x = y?=w415:bool)
        n200 = case shown="True" w415 {
          tunnel: [w424 w436] -> w420
          tunnel: w419 -> [w424 w431]
          tunnel: w418 -> [_ w430]
          frame False {
          }
          frame True {
            n201 = Bundle By Name(cluster=T5 {"Color"=0, "Pen"={"Width"=2, "Style"=enum."Solid"}} ("Style"), "Color"="Line Color", "Pen.Width"="Line Width", "Pen.Style"="Line Type") -> (w425:T5)
            n202 = case shown="\"Line\", Default" "Tool Box" {
              tunnel: [w440 w445 w450] -> w433
              tunnel: w425 -> [w437 w442 w447]
              frame "Line", Default {
                n203 = call "Set Style.vi"("Style"=w437, "Graphic in"=refnum<class "Line.lvclass"> refnum ("Line.lvclass")) -> ("Graphic out"=w438:refnum<class "Line.lvclass">)  [unwired: 8 in, 1 out]
                n204 = call "Set Border.vi"("Scalable Border.lvclass"=refnum<class "Line Border.lvclass"> refnum ("Line Border.lvclass"), "Graphic in"=w438) -> ("Graphic out"=w440:refnum<class "Line.lvclass">)  [unwired: 8 in, 1 out]
              }
              frame "Rectangle" {
                n205 = call "Set Style.vi"("Style"=w442, "Graphic in"=refnum<class "Rectangle.lvclass"> refnum ("Rectangle.lvclass")) -> ("Graphic out"=w443:refnum<class "Rectangle.lvclass">)  [unwired: 8 in, 1 out]
                n206 = call "Set Border.vi"("Scalable Border.lvclass"=refnum<class "Rectangle Border.lvclass"> refnum ("Rectangle Border.lvclass"), "Graphic in"=w443) -> ("Graphic out"=w445:refnum<class "Rectangle.lvclass">)  [unwired: 8 in, 1 out]
              }
              frame "Triangle" {
                n207 = call "Set Style.vi"("Style"=w447, "Graphic in"=refnum<class "Triangle.lvclass"> refnum ("Triangle.lvclass")) -> ("Graphic out"=w448:refnum<class "Triangle.lvclass">)  [unwired: 8 in, 1 out]
                n208 = call "Set Border.vi"("Scalable Border.lvclass"=refnum<class "Rectangle Border.lvclass"> refnum ("Rectangle Border.lvclass"), "Graphic in"=w448) -> ("Graphic out"=w450:refnum<class "Triangle.lvclass">)  [unwired: 8 in, 1 out]
              }
            }
            n209 = call-dynamic "Mouse Down.vi"("Point"=w430, "Graphic in"=w433) -> ("Graphic out"=w432:refnum<class "Graphic.lvclass">)  [unwired: 8 in, 1 out]
            n210 = Bundle By Name(cluster=w431, "Status"=Status."Drawing", "Drawing Graphic"=w432) -> (w436:T11)
          }
        }
        n211 = call <vilib>:"Add State(s) to Queue__JKI_lib_State_Machine.vi"("State(s) in (\"\")"=w423) -> ("States Out"=w422:string)  [unwired: 14 in]
      }
      frame "Modify Selected Graphic" {
        n212 = Unbundle By Name(w454) -> ("Canvas"=w453:refnum<class "Canvas.lvclass">)
        n213 = call "Delete Active Graphic.vi"("Canvas in"=w453) -> ("Canvas out"=w452:refnum<class "Canvas.lvclass">)  [unwired: 9 in, 1 out]
        n214 = Bundle By Name(cluster=w454, "Status"=Status."Modify", "Canvas"=w452) -> (w456:T11)
        n215 = call <vilib>:"Add State(s) to Queue__JKI_lib_State_Machine.vi"("State(s) in (\"\")"=w459) -> ("States Out"=w458:string)  [unwired: 14 in]
      }
      frame "Check Click In Border" {
        n216 = Unbundle By Name(w470) -> ("Canvas"=w469:refnum<class "Canvas.lvclass">, "MouseDown Coords"=w466:T10)
        n217 = call "Check Mouse In Border Focus.vi"("error in (no error)"=w465, "MousePoint"=w466, "Canvas in"=w469) -> ("error out"=w464:errorcluster, "In Border Focus"=w463:bool, "Canvas out"=w467:refnum<class "Canvas.lvclass">)  [unwired: 6 in]
        n218 = Bundle By Name(cluster=w470, "Canvas"=w467) -> (w468:T11)
        n219 = Select(t="Modify Selected Graphic", s=w463, f="Draw New Graphic") -> (s? t:f=w460:string)
        n220 = call <vilib>:"Add State(s) to Queue__JKI_lib_State_Machine.vi"("State(s) in (\"\")"=w472, "State(s) at Back (\"\")"=w460) -> ("States Out"=w471:string)  [unwired: 13 in]
      }
      frame "Check Click On Graphic" {
        n221 = Unbundle By Name(w479) -> ("Canvas"=w478:refnum<class "Canvas.lvclass">, "MouseDown Coords"=w477:T10)
        n222 = call "Active Graphic On Click.vi"("MousePoint"=w477, "Canvas in"=w478) -> ("Find?"=w473:bool, "Canvas out"=w475:refnum<class "Canvas.lvclass">)  [unwired: 7 in, 1 out]
        n223 = case shown="True" w473 {
          tunnel: w475 -> [w484 w486]
          tunnel: [w483 w485] -> w474
          frame False {
            n224 = call "Cancel Active Graphic On Click.vi"("Canvas in"=w484) -> ("Canvas out"=w483:refnum<class "Canvas.lvclass">)  [unwired: 9 in, 1 out]
          }
          frame True {
            n225 = call "Draw Border On Active Graphic.vi"("Canvas in"=w486) -> ("Canvas out"=w485:refnum<class "Canvas.lvclass">)  [unwired: 9 in, 1 out]
          }
        }
        n226 = Bundle By Name(cluster=w479, "Canvas"=w474) -> (w476:T11)
        n227 = call <vilib>:"Add State(s) to Queue__JKI_lib_State_Machine.vi"("State(s) in (\"\")"=w482) -> ("States Out"=w481:string)  [unwired: 14 in]
      }
    }
  }
